vi "mag_globals.vi"() -> ()   [LabVIEW 2014]
panel:
  in  "Calibrate scaling":dbl[](array[numeric])=[1.0, 1.0]
  # "Map calibration scale and offset to well-scaled states.  At one point I was using [1e-6, 1], but right now Ks and r bias have similar magnitudes."
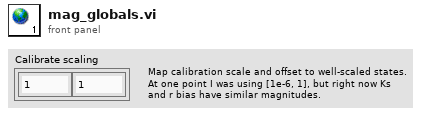
[diagram p1: front panel]
diagram:
